vi "primary control loop.vi"(8 "worker pool reference":T18, 9 "fault fifo":refnum<k33>, 10 "cmd fifo":refnum<k33>, 11 "engine out":T1={"timed loop timer source"={"Processor"=-2, "Priority"=0, "timing source dt"=0, "timer source"=refnum}, "control loop data"={"engine tag bus"={"Double"=[], "Single"=[], "I64"=[], "I32"=[], "I16"=[], "I8"=[], "U64"=[], "U32"=[], "U16"=[], "U8"=[], "Boolean"=[], "String"=[], "Array of Double"=[], "Array of Single"=[], "Array of I64"=[], "Array of I32"=[], "Array of I16"=[], "Array of I8"=[], "Array of U64"=[], "Array of U32"=[], "Array of U16"=[], "Array of U8"=[], "Array of Boolean"=[], "Array of String"=[]}, "engine schedule"={"module run flags"=[], "decimation schedule"={"decimations"=[], "offsets"=[]}}, "module information"=[]}, "status reporting"={"late? index (bool)"=-1, "late count index (U32)"=-1, "dt (ns) index (U64)"=-1}} {"control loop data"."module information"."GUID"."Lo" format="%.0x"; "control loop data"."module information"."GUID"."Hi" format="%.0x"}) -> (0 "error out":errorcluster, 2 "desired state":T21, 3 "engine out":T1={"timed loop timer source"={"Processor"=-2, "Priority"=0, "timing source dt"=0, "timer source"=refnum}, "control loop data"={"engine tag bus"={"Double"=[], "Single"=[], "I64"=[], "I32"=[], "I16"=[], "I8"=[], "U64"=[], "U32"=[], "U16"=[], "U8"=[], "Boolean"=[], "String"=[], "Array of Double"=[], "Array of Single"=[], "Array of I64"=[], "Array of I32"=[], "Array of I16"=[], "Array of I8"=[], "Array of U64"=[], "Array of U32"=[], "Array of U16"=[], "Array of U8"=[], "Array of Boolean"=[], "Array of String"=[]}, "engine schedule"={"module run flags"=[], "decimation schedule"={"decimations"=[], "offsets"=[]}}, "module information"=[]}, "status reporting"={"late? index (bool)"=-1, "late count index (U32)"=-1, "dt (ns) index (U64)"=-1}} {"control loop data"."module information"."GUID"."Lo" format="%.0x"; "control loop data"."module information"."GUID"."Hi" format="%.0x"})   [LabVIEW 2013, in "main engine.lvlib"]
uses:
  main engine/main engine.lvlib
  engine state.ctl
  worker library/worker comms.ctl
  worker library/worker commands.ctl
  worker library/request fifos.ctl
  worker library/recovery request.ctl
  <vilib>/NI/Tag Bus Module Framework/runtime/TBM module execution interface.lvclass
  <vilib>/NI/Tag Bus Module Framework/module configuration/TBM module configuration.lvclass
  worker library/response fifos.ctl
  worker library/recovery response.ctl
  rt fault.ctl
  <vilib>/NI/Tag Bus Module Framework/runtime/error classification.ctl
  Engine Data.ctl
  <vilib>/NI/Module Timing Source/timing source/TBM timing source.lvclass
  timed loop timing sources.ctl
  control loop data.ctl
  <vilib>/NI/Tag Bus/table/data table.ctl
  engine run schedule.ctl
  engine decimation schedule.ctl
  full module data.ctl
  module run state.ctl
  async executor/asynchronous executor reference.ctl
  async executor/message to executor.ctl
  async command notification.ctl
  async error info.ctl
  <vilib>/NI/Tag Bus/buffer exchange/buffer reference.ctl
  <vilib>/NI/Configuration Framework/serializable configuration/Numeric GUID.ctl
  module method data.ctl
  <vilib>/NI/Tag Bus/table/transfer specification.ctl
  <vilib>/NI/Tag Bus/tag/Data Type.ctl
  fault handling spec.ctl
  Configuration/Error Actions.ctl
  status reporting data.ctl
  <vilib>/Platform/TimedLoop/XDataNode/timing_clust.ctl
  <vilib>/Platform/TimedLoop/XDataNode/nitl_modes.ctl
  <vilib>/Platform/TimedLoop/XDataNode/wakeup.ctl
  time information.ctl
  <vilib>/NI/Tag Bus/table/transfer table data.vi
  decimate.vi
  fault and error bookkeeping.vi
  report timing.vi
  wait for recovered modules.vi
  <vilib>/NI/Tag Bus/table/write data element.vi
  <vilib>/NI/Tag Bus/table/data polymorphs/write one/write I32.vi
  perform asynchronous fault handling.vi
  perform fault handling.vi
  <vilib>/NI/Tag Bus/table/data polymorphs/write one/write Boolean.vi
  <vilib>/NI/Tag Bus/table/data polymorphs/write one/write U32.vi
  <vilib>/NI/Tag Bus/table/data polymorphs/write one/write U64.vi
  rt swap object in dvr.vi
  worker library/request recovery.vi
  async executor/input data method.vi
  async executor/process data method.vi
  async executor/output data method.vi
  <vilib>/platform/TimedLoop/XDataNode/XDataNode.xnode
  <vilib>/Platform/TimedLoop/XDataNode/XDNodeRunTimeDep.lvlib
  <vilib>/NI/Tag Bus/table/data table.lvlib
  <vilib>/NI/Tag Bus/buffer exchange/tag bus buffer exchange.lvlib
  async executor/async executor.lvlib
  <vilib>/NI/Tag Bus/tag/tag descriptor.lvclass
  Configuration/Standard Engine Configuration.lvclass
  <vilib>/NI/Configuration Framework/serializable configuration/NISE_CEF_serializable configuration.lvclass
  worker library/worker pool.lvlib
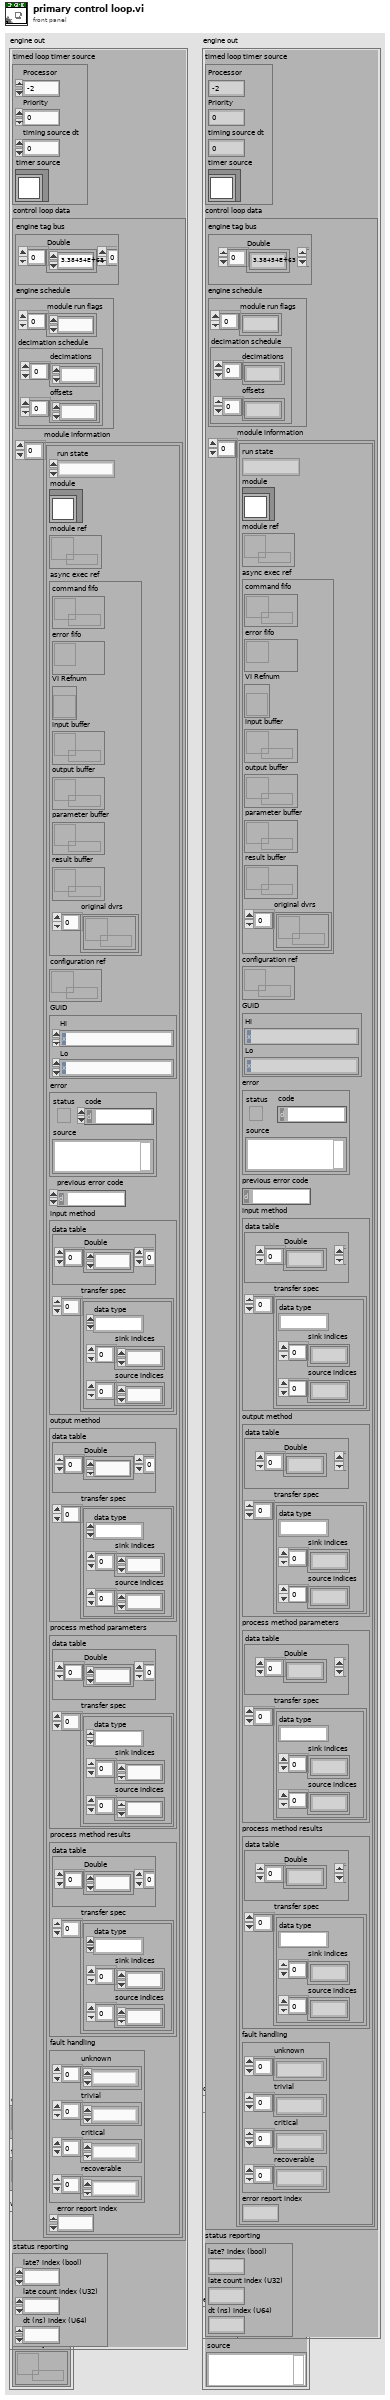
[diagram p1: front panel]
types:
  T1 = typedef "main engine.lvlib/Engine Data.ctl" = cluster{"timed loop timer source":T2, "control loop data":T3, "status reporting":T17}
  T2 = typedef "main engine.lvlib/timed loop timing sources.ctl" = cluster{"Processor":i32, "Priority":i32, "timing source dt":u32, "timer source":refnum<class "TBM timing source.lvclass">}
  T3 = typedef "main engine.lvlib/control loop data.ctl" = cluster{"engine tag bus":T4, "engine schedule":T5, "module information":T7[]}
  T4 = typedef "tag bus.lvlib/data table.lvlib/data table.ctl" = cluster{"Double":dbl[], "Single":sgl[], "I64":i64[], "I32":i32[], "I16":i16[], "I8":i8[], "U64":u64[], "U32":u32[], "U16":u16[], "U8":u8[], "Boolean":bool[], "String":string[], "Array of Double":cluster{"DBL Array":dbl[]}[], "Array of Single":cluster{"SGL Array":sgl[]}[], "Array of I64":cluster{"I64 Array":i64[]}[], "Array of I32":cluster{"I32 Array":i32[]}[], "Array of I16":cluster{"I16 Array":i16[]}[], "Array of I8":cluster{"I8 Array":i8[]}[], "Array of U64":cluster{"U64 Array":u64[]}[], "Array of U32":cluster{"U32 Array":u32[]}[], "Array of U16":cluster{"U16 Array":u16[]}[], "Array of U8":cluster{"U8 Array":u8[]}[], "Array of Boolean":cluster{"Boolean Array":bool[]}[], "Array of String":cluster{"String Array":string[]}[]}
  T5 = typedef "main engine.lvlib/engine run schedule.ctl" = cluster{"module run flags":u8[], "decimation schedule":T6}
  T6 = typedef "main engine.lvlib/engine decimation schedule.ctl" = cluster{"decimations":u16[], "offsets":u16[]}
  T7 = typedef "main engine.lvlib/full module data.ctl" = cluster{"run state":T8, "module":refnum<class "TBM module execution interface.lvclass">, "module ref":refnum<data-value>, "async exec ref":T9, "configuration ref":refnum<data-value>, "GUID":T11, "error":errorcluster, "previous error code":i32, "input method":T12, "output method":T12, "process method parameters":T12, "process method results":T12, "fault handling":T15, "error report index ":i32}
  T8 = typedef "main engine.lvlib/module run state.ctl" = enum16{"sync", "async"}
  T9 = typedef "async executor.lvlib/asynchronous executor reference.ctl" = cluster{"command fifo":refnum<k33>, "error fifo":refnum<k33>, "VI Refnum":refnum<vi>, "input buffer":refnum<k33>, "output buffer":refnum<k33>, "parameter buffer":refnum<k33>, "result buffer":refnum<k33>, "original dvrs":T10[]}
  T10 = typedef "tag bus buffer exchange.lvlib/buffer reference.ctl" = refnum<data-value>
  T11 = typedef "NISE_CEF_serializable configuration.lvclass/Numeric GUID.ctl" = cluster{"Hi":u64, "Lo":u64}
  T12 = typedef "main engine.lvlib/module method data.ctl" = cluster{"data table":T4, "transfer spec":T13[]}
  T13 = typedef "tag bus.lvlib/data table.lvlib/transfer specification.ctl" = cluster{"data type":T14, "sink indices":i32[], "source indices":i32[]}
  T14 = typedef "tag bus.lvlib/tag descriptor.lvclass/Data Type.ctl" = enum16{"Double", "Single", "I64", "I32", "I16", "I8", "U64", "U32", "U16", "U8", "Boolean", "String", "Array of Double", "Array of Single", "Array of I64", "Array of I32", "Array of I16", "Array of I8", "Array of U64", "Array of U32", "Array of U16", "Array of U8", "Array of Boolean", "Array of String"}
  T15 = typedef "main engine.lvlib/fault handling spec.ctl" = cluster{"unknown":T16[], "trivial":T16[], "critical":T16[], "recoverable":T16[]}
  T16 = typedef "Standard Engine Configuration.lvclass/Error Actions.ctl" = enum16{"Clear", "Notify", "Stop Component", "Stop Engine", "Safe State", "Attempt Recovery"}
  T17 = typedef "main engine.lvlib/status reporting data.ctl" = cluster{"late? index (bool)":i32, "late count index (U32)":i32, "dt (ns) index (U64)":i32}
  T18 = typedef "worker pool.lvlib/worker comms.ctl" = cluster{"command fifo":refnum<k33>, "request fifos":T19, "response fifos":T20}
  T19 = typedef "worker pool.lvlib/request fifos.ctl" = cluster{"recovery":refnum<k33>}
  T20 = typedef "worker pool.lvlib/response fifos.ctl" = cluster{"recovery":refnum<k33>}
  T21 = typedef "main engine.lvlib/engine state.ctl" = enum16{"idle", "configured", "running", "safe state", "exit"}
  T22 = typedef "main engine.lvlib/time information.ctl" = cluster{"ns since last call":u64, "finished late?":bool, "late count":u32, "iterations":u64}
  T23 = typedef "XDNodeRunTimeDep.lvlib/timing_clust.ctl" = cluster{"Expected End [f-1]":u64, "Actual End [f-1]":u64, "Finished Late? [f-1]":bool, "Expected End [i-1]":u64, "Actual End [i-1]":u64, "Finished Late? [i-1]":bool, "Expected Start [i]":u64, "Actual Start [i]":u64, "Expected Start [f]":u64, "Actual Start [f]":u64, "Source Name":string, "Structure Name":string, "Period":i64, "Deadline":i64, "Offset":i64, "Start":i64, "Priority":i32, "Timeout":i32, "Mode":T24, "Wakeup Reason":T25, "Error":errorcluster, "Source Type":string, "Secondary Source Type":string, "Global End Time":u64, "Global Start Time":u64, "Frame Duration":u64, "Iteration Duration":u64, "Assigned CPU":i32, "I/O Scan Engine Mode":u32}
  T24 = typedef "XDNodeRunTimeDep.lvlib/nitl_modes.ctl" = enum32{"No Change", "Process missed periods, maintain original phase", "Discard missed periods, maintain original phase", "Process missed periods, ignore original phase", "Discard missed periods, ignore original phase"}
  T25 = typedef "XDNodeRunTimeDep.lvlib/wakeup.ctl" = enum32{"Normal", "Aborted", "Asynchronous wakeup", "Timing source error", "Timed loop error", "Timeout"}
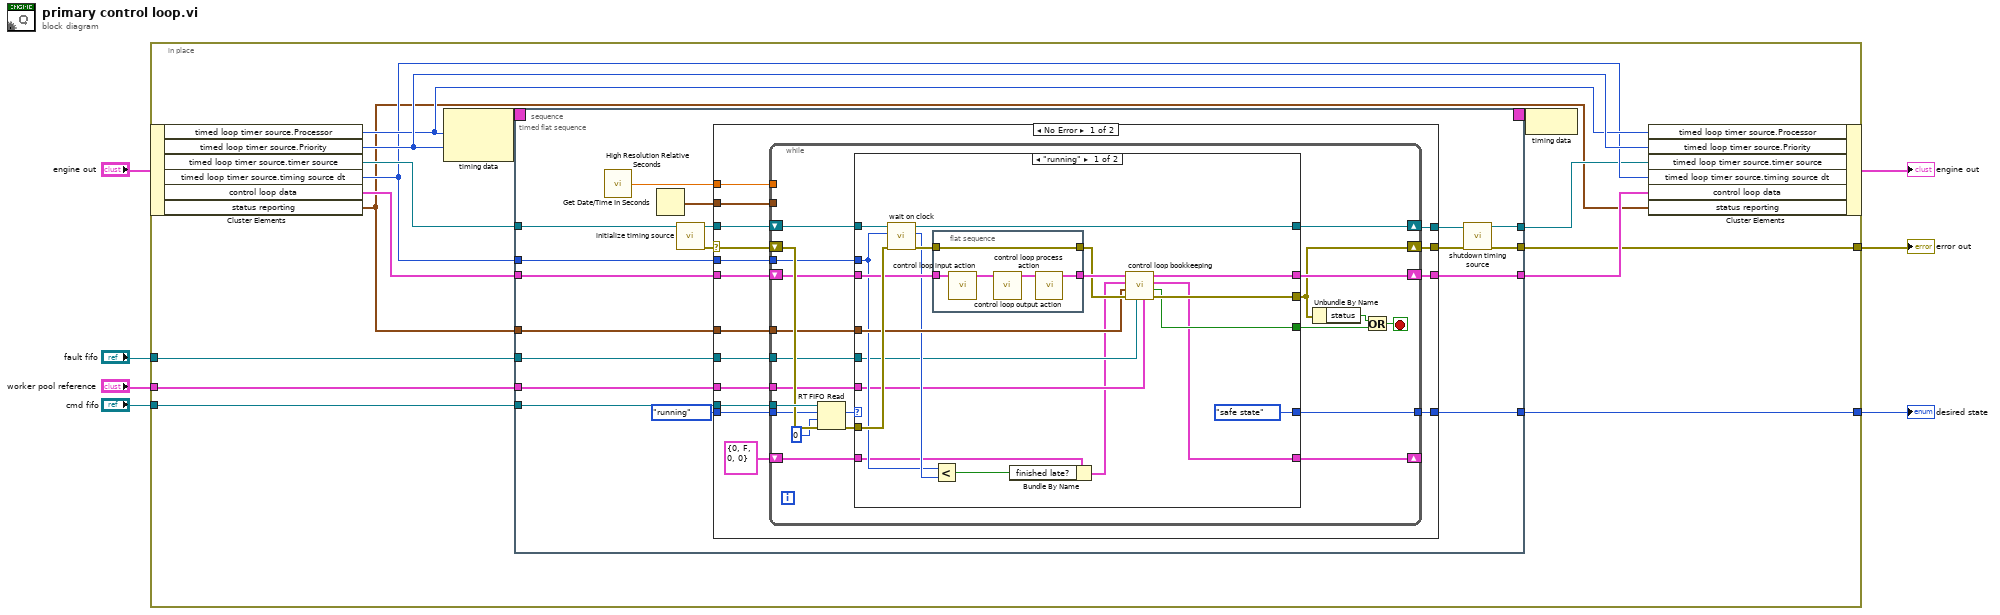
[diagram p0: block diagram]
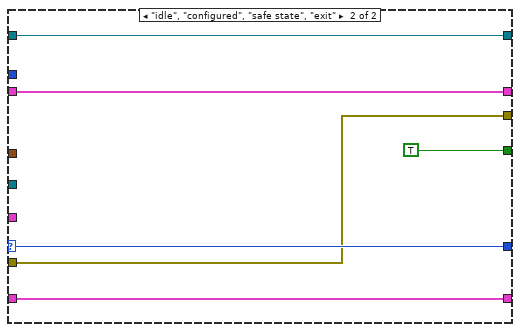
[diagram p2: hidden frame]
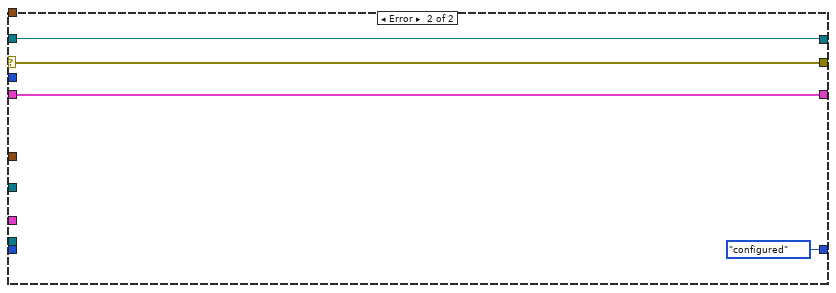
[diagram p3: hidden frame]
diagram:
  n1 = in-place {
    in-place-border: [w13] -> w5
    in-place-border: "cmd fifo" -> [w12]
    in-place-border: "fault fifo" -> [w11]
    in-place-border: "worker pool reference" -> [w10]
    in-place-border: [w9] -> w1
    n2 = in-place-cluster #1("engine out") -> ("timed loop timer source.Processor"=w17:i32, "timed loop timer source.Priority"=w18:i32, "timed loop timer source.timer source"=w20:refnum<class "TBM timing source.lvclass">, "timed loop timer source.timing source dt"=w16:u32, "control loop data"=w19:T3, "status reporting"=w8:T17)
    n3 = node-c288(w17, w18) -> (w22:T23)
    n4 = timed-sequence {
      timing: w22 -> [_]
      timing-out: [_] -> w21
      tunnel: w20 -> [w33]
      tunnel: w19 -> [w28]
      tunnel: w16 -> [w32]
      tunnel: [w31] -> w15
      tunnel: [w30] -> w13
      tunnel: [w29] -> w14
      tunnel: w12 -> [w27]
      tunnel: w11 -> [w26]
      tunnel: w10 -> [w25]
      tunnel: [w24] -> w9
      tunnel: w8 -> [w23]
      n5 = timed-flat-sequence {
        tunnel: w33 -> [w51]
        tunnel: w32 -> [w49]
        tunnel: [w42] -> w31
        tunnel: [w44] -> w30
        tunnel: [w46] -> w29
        tunnel: w28 -> [w45]
        tunnel: w27 -> [w41]
        tunnel: w26 -> [w40]
        tunnel: w25 -> [w39]
        tunnel: [w37] -> w24
        tunnel: w23 -> [w34]
        n6 = call <vilib>:"High Resolution Relative Seconds.vi"() -> ("relative seconds"=w35:dbl)
        n7 = Get Date/Time In Seconds() -> (seconds since 1Jan1904=w36:timestamp)
        n8 = call-dynamic "initialize timing source.vi"("timing source in"=w51) -> ("error out"=w50:errorcluster, "timing source out"=w48:refnum<class "TBM timing source.lvclass">)  [unwired: 9 in]
        n9 = case shown="No Error" w50 {
          selector: w50 -> [w65 w122]
          tunnel: w49 -> [w56 _]
          tunnel: [w66 w123] -> w43
          tunnel: w48 -> [w67 w123]
          tunnel: [w64 w122] -> w47
          tunnel: [w62 w121] -> w46
          tunnel: w45 -> [w63 w121]
          tunnel: w41 -> [w61 _]
          tunnel: w40 -> [w60 _]
          tunnel: w39 -> [w59 _]
          tunnel: engine_state."running" ("element") -> [w58 _]
          tunnel: [w57 engine_state."configured"] -> w37
          tunnel: w36 -> [w55 _]
          tunnel: w35 -> [w54 _]
          tunnel: w34 -> [w53 _]
          frame No Error {
            n10 = while {
              shift-right: [w79] -> w66
              shift-left: w67 -> [w80]
              shift-right: [w72] -> w64
              shift-left: w65 -> [w87]
              shift-right: [w77] -> w62
              shift-left: w63 -> [w78]
              tunnel: w61 -> [w88]
              tunnel: w60 -> [w76]
              tunnel: w59 -> [w74]
              tunnel: w58 -> [w85]
              tunnel: [w82] -> w57
              tunnel: w56 -> [w75]
              tunnel: w55 -> [_]
              tunnel: w54 -> [_]
              tunnel: w53 -> [w70]
              shift-right: [w68] -> _
              shift-left: T22 {"ns since last call"=0, "finished late?"=FALSE, "late count"=0, "iterations"=0} ("time data") -> [w69]
              stop <- w73 stop-if-true
              n11 = RT FIFO Read(0:w88, 1:w85, 2:0 ("timeout in ms (0)"), 3:w87) -> (9:w84:T21, 11:w83:errorcluster)  [unwired: 3 out]
              n12 = case shown="\"running\"" w84 {
                selector: w84 -> [_ w119]
                tunnel: w83 -> [w107 w118]
                tunnel: [engine_state."safe state" w119] -> w82
                tunnel: [w97 w118] -> w72
                tunnel: [w96 TRUE] -> w81
                tunnel: w80 -> [w108 w116]
                tunnel: [w106 w116] -> w79
                tunnel: w78 -> [w105 w115]
                tunnel: [w104 w115] -> w77
                tunnel: w76 -> [w94 _]
                tunnel: w75 -> [w98 _]
                tunnel: w74 -> [w93 _]
                tunnel: w70 -> [w100 _]
                tunnel: w69 -> [w92 w114]
                tunnel: [w91 w114] -> w68
                frame "running" {
                  n13 = call-dynamic "wait on clock.vi"("error in"=w107, "dt"=w98, "timing source in"=w108) -> ("error out"=w102:errorcluster, "ticks since last call"=w99:u32, "timing source out"=w106:refnum<class "TBM timing source.lvclass">)  [unwired: 6 in]
                  n14 = flat-sequence {
                    tunnel: w105 -> [w111]
                    tunnel: [w110] -> w103
                    tunnel: w102 -> [w109]
                    tunnel: [w109] -> w101
                    frame #0 {
                      n15 = call "control loop input action.vi"("control loop data in"=w111) -> ("control loop data out"=w113:T3)  [unwired: 10 in]
                      n16 = call "control loop process action.vi"("control loop data in"=w113) -> ("control loop data out"=w112:T3)  [unwired: 10 in]
                      n17 = call "control loop output action.vi"("control loop data in"=w112) -> ("control loop data out"=w110:T3)  [unwired: 10 in]
                    }
                  }
                  n18 = Less?(x=w98, y=w99) -> (x < y?=w89:bool)
                  n19 = Bundle By Name(cluster=w92, "finished late?"=w89) -> (w90:T22)
                  n20 = call "control loop bookkeeping.vi"("worker pool reference"=w93, "fault fifo"=w94, "engine error in"=w101, "status reporting in"=w100, "time data in"=w90, "control loop data in"=w103) -> ("engine error out"=w97:errorcluster, "safe state?"=w96:bool, "time data out"=w91:T22, "control loop data out"=w104:T3)  [unwired: 2 in]
                }
                frame "idle", "configured", "safe state", "exit" {
                }
              }
              n21 = Unbundle By Name(w72) -> ("status"=w71:bool)
              n22 = Or(x=w71, y=w81) -> (x .or. y?=w73:bool)
            }
          }
          frame Error {
          }
        }
        n23 = call-dynamic "shutdown timing source.vi"("error in"=w47, "timing source in"=w43) -> ("error out"=w44:errorcluster, "timing source out"=w42:refnum<class "TBM timing source.lvclass">)  [unwired: 8 in]
      }
    }
    n24 = node-c288(w21) -> ()
    n25 = in-place-cluster #1("timed loop timer source.Processor"=w17, "timed loop timer source.Priority"=w18, "timed loop timer source.timer source"=w15, "timed loop timer source.timing source dt"=w16, "control loop data"=w14, "status reporting"=w8) -> (→"engine out":T1)
  }
  "desired state" <- w1
  "error out" <- w5
